vi "MGI Get LB Row Str[].vi"(7 "MGI Error Reporter Base In":refnum<class "MGI Error Reporter Base.lvclass">, 11 "MGI ERD Time and Count Storage In":refnum<class "MGI ERD LB Row Time and Count.lvclass">) -> (2 "String[col]":string[](array[string]))   [LabVIEW 2020, in "MGI ERD LB Row Time and Count.lvclass"]
doc: "Authored by Shawn Walpole\nsupport@mooregoodideas.com\nwww.mooregoodideas.com\n\nCopyright (c) 2013, Moore Good Ideas, Inc.\n\nAll rights reserved.\n\nRedistribution and use in source and binary forms, with or without modification, are permitted provided that the following conditions are met:\n\n * Redistributions of source code must retain the above copyright notice, this list of conditions and the following disclaimer.\n * Redistributions in binary form must reproduce the above copyright notice, this list of conditions and the following disclaimer in the documentation and/or other materials provided with the distribution.\n * Neither the name of Moore Good Ideas, Inc. nor the names of its contributors may be used to endorse or promote products derived from this software without specific prior written permission.\n\nTHIS SOFTWARE IS PROVIDED BY THE COPYRIGHT HOLDERS AND CONTRIBUTORS \"AS IS\" AND ANY EXPRESS OR IMPLIED WARRANTIES, INCLUDING, BUT NOT LIMITED TO, THE IMPLIED WARRANTIES OF MERCHANTABILITY AND FITNESS FOR A PARTICULAR PURPOSE ARE DISCLAIMED. IN NO EVENT SHALL THE COPYRIGHT OWNER OR CONTRIBUTORS BE LIABLE FOR ANY DIRECT, INDIRECT, INCIDENTAL, SPECIAL, EXEMPLARY, OR CONSEQUENTIAL DAMAGES (INCLUDING, BUT NOT LIMITED TO, PROCUREMENT OF SUBSTITUTE GOODS OR SERVICES; LOSS OF USE, DATA, OR PROFITS; OR BUSINESS INTERRUPTION) HOWEVER CAUSED AND ON ANY THEORY OF LIABILITY, WHETHER IN CONTRACT, STRICT LIABILITY, OR TORT (INCLUDING NEGLIGENCE OR OTHERWISE) ARISING IN ANY WAY OUT OF THE USE OF THIS SOFTWARE, EVEN IF ADVISED OF THE POSSIBILITY OF SUCH DAMAGE."
uses:
  <userlib>/_MGI/Error Reporter/MGI Error Reporter Dialog/MGI ERD LB Row Time and Count/MGI ERD LB Row Time and Count.lvclass
  <userlib>/_MGI/Error Reporter/MGI Error Reporter Base/MGI Error Reporter Base.lvclass
  C:/Program Files/National Instruments/LabVIEW 2020/user.lib/_MGI/Error Reporter/MGI Error Reporter Dialog/MGI ERD LB Row Base/MGI ERD LB Row Base.lvclass
  <userlib>/_MGI/Error Reporter/MGI Error Reporter Dialog/MGI ERD LB Row Time and Count/MGI ERD LB Row Time and Count.lvclass/MGI ERD LB Row Time and Count.ctl
  <userlib>/_MGI/Error Reporter/MGI Error Reporter Dialog/MGI ERD LB Row Base/MGI ERD LB Row Base.lvclass
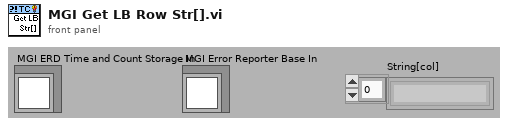
[diagram p1: front panel]
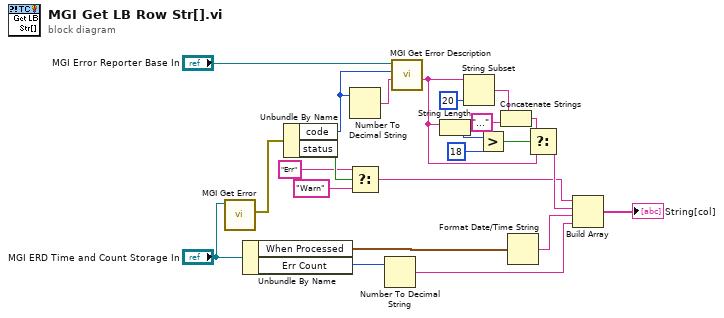
[diagram p0: block diagram]
diagram:
  n1 = call <userlib>:"MGI Get Error.vi"("MGI ERD LB Row Base in"="MGI ERD Time and Count Storage In") -> ("error"=w1:errorcluster)  [unwired: 10 out]
  n2 = Unbundle By Name("MGI ERD Time and Count Storage In") -> ("When Processed"=w9:timestamp, "Err Count"=w3:i32)
  n3 = Unbundle By Name(w1) -> ("code"=w22:i32, "status"=w21:bool)
  n4 = Number To Decimal String(number=w22) -> (decimal integer string=w12:string)  [unwired: 1 out]
  n5 = Select(t="Err", s=w21, f="Warn") -> (s? t:f=w8:string)
  n6 = Number To Decimal String(number=w3) -> (decimal integer string=w11:string)  [unwired: 1 out]
  n7 = call <userlib>:"MGI Get Error Description.vi"("Default Description"=w12, "Error Code"=w22, "MGI Error Reporter Base In"="MGI Error Reporter Base In") -> ("Error Name"=w23:string)  [unwired: 8 out]
  n8 = String Length(string=w23) -> (length=w13:i32)
  n9 = String Subset(string=w23, length (rest)=20 ("y")) -> (substring=w18:string)  [unwired: 1 out]
  n10 = Greater?(x=w13, y=18) -> (0:w15:bool)
  n11 = Concatenate Strings(w18, "...") -> (w19:string)
  n12 = Format Date/Time String(seconds (now)=w9) -> (date/time string=w10:string)  [unwired: 2 out]
  n13 = Select(t=w19, s=w15, f=w23) -> (s? t:f=w16:string)
  n14 = Build Array(w8, w16, w10, w11) -> (→"String[col]":string[])
